vi "Tosca-Initialize Imaging.vi"(0 "Tosca":refnum<class "Parameters.lvclass">, 11 "error in (no error)":errorcluster) -> (4 "Tosca out":refnum<class "Parameters.lvclass">, 15 "error out":errorcluster)   [LabVIEW 2020]
uses:
  Classes/Parameters/Parameters.lvclass
  Classes/Parameters/Parameters.lvclass/Parameters.ctl
  Classes/Parameters/Read DAQ.vi
  Classes/Parameters/Read Imaging.vi
  Classes/Parameters/Write DAQ.vi
  Classes/Parameters/Write Imaging.vi
  Classes/Parameters/Read mode.vi
  Tosca-2P-Globals.vi
  Classes/State/Set AO Sampling Rate.vi
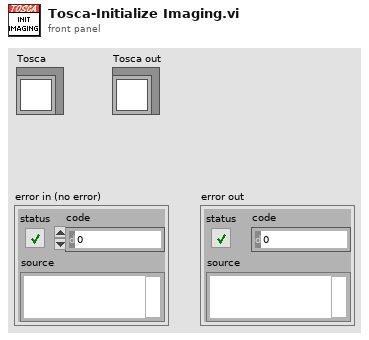
[diagram p1: front panel]
types:
  T1 = typedef "Tosca-Imaging Mode.ctl" = enum16{"Off", "Widefield", "Two-photon"}
  T2 = typedef "Parameters.lvclass/DAQ.ctl" = cluster{"AO Fs (Hz)":dbl, "DO Fs (Hz)":dbl, "Poll Rate (Hz)":dbl, "Baseline (s)":dbl}
  T3 = typedef "Tosca-Imaging.ctl" = cluster{"mode":T1, "FrameRateHz":dbl, "use AO":bool, "destination":string}
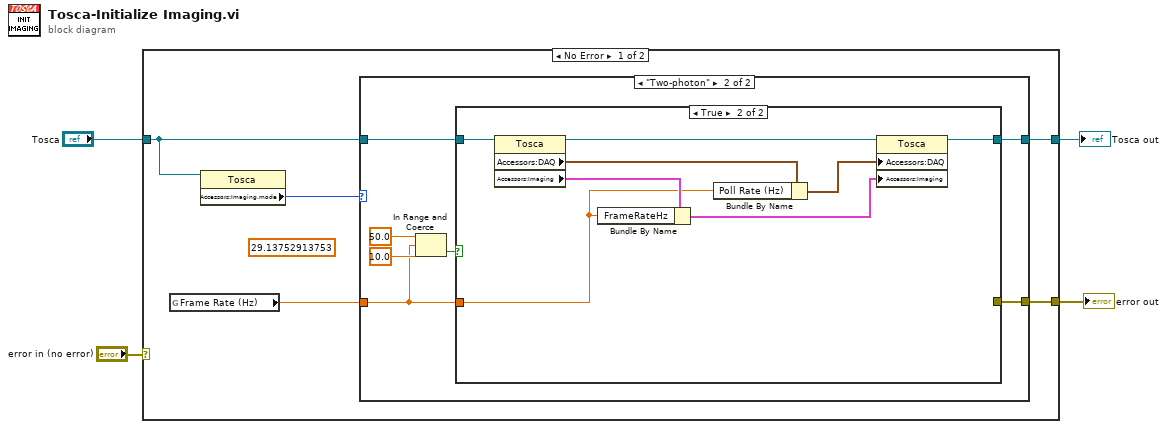
[diagram p0: block diagram]
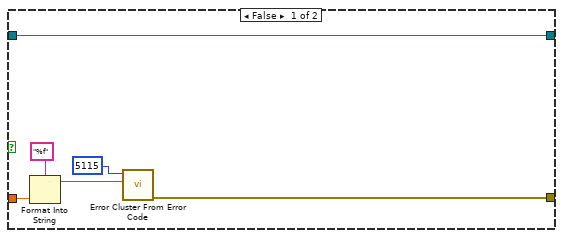
[diagram p3: hidden frame]
diagram:
  n1 = case shown="No Error" "error in (no error)" {
    selector: "error in (no error)" -> [_ w32]
    tunnel: [w8 w32] -> w3
    tunnel: [w9 w33] -> w1
    tunnel: "Tosca" -> [w6 w33]
    frame No Error {
      (unwired) 29.13752913753 ("Frame Rate (Hz)")
      n2 = global read "Tosca-2P-Globals.vi" "Frame Rate (Hz)"() -> (w7:dbl)
      n3 = property class="Tosca"(reference=w6) -> ("Accessors:Imaging.mode"=w5:T1)  [unwired: 1 in, 2 out]
      n4 = case shown="\"Two-photon\"" w5 {
        tunnel: [w10 w16] -> w9
        tunnel: w6 -> [w10 w17]
        tunnel: w7 -> [_ w11]
        tunnel: [_ w12] -> w8
        frame "Off", Default {
        }
        frame "Two-photon" {
          n5 = In Range and Coerce(upper limit=50.0, x=w11, lower limit=10.0) -> (In Range?=w13:bool)  [unwired: 1 out]
          n6 = case shown="True" w13 {
            tunnel: w17 -> [w20 w31]
            tunnel: [w20 w27] -> w16
            tunnel: w11 -> [w22 w24]
            tunnel: [w19 _] -> w12
            frame False {
              n7 = Format Into String(format string="%f", w22) -> (resulting string=w21:string)  [unwired: 2 in, 1 out]
              n8 = call <vilib>:"Error Cluster From Error Code.vi"("error message (\"\")"=w21, "error code (0)"=5115) -> ("error out"=w19:errorcluster)  [unwired: 7 in]
            }
            frame True {
              n9 = property class="Tosca"(reference=w31) -> (reference out=w29:refnum<class "Parameters.lvclass">, "Accessors:DAQ"=w30:T2, "Accessors:Imaging"=w26:T3)  [unwired: 1 in, 1 out]
              n10 = Bundle By Name(cluster=w26, "FrameRateHz"=w24) -> (w25:T3)
              n11 = Bundle By Name(cluster=w30, "Poll Rate (Hz)"=w24) -> (w28:T2)
              n12 = property class="Tosca"(reference=w29, "Accessors:DAQ"=w28, "Accessors:Imaging"=w25) -> (reference out=w27:refnum<class "Parameters.lvclass">)  [unwired: 1 in, 1 out]
            }
          }
        }
      }
    }
    frame Error {
    }
  }
  "Tosca out" <- w1
  "error out" <- w3
